vi "(Depricated) Poll Stepper Enable.vi"(8 "error in (no error)":errorcluster, 11 "cRIO-CO2 in":refnum<class "cRIO-CO2.lvclass">) -> (0 "error out":errorcluster, 3 "cRIO-CO2 out":refnum<class "cRIO-CO2.lvclass">)   [LabVIEW 2015]
uses:
  cRIO-CO2 Messages/Launch Stepper Msg/Launch Syringe Stepper Msg.lvclass
  cRIO-CO2.lvclass
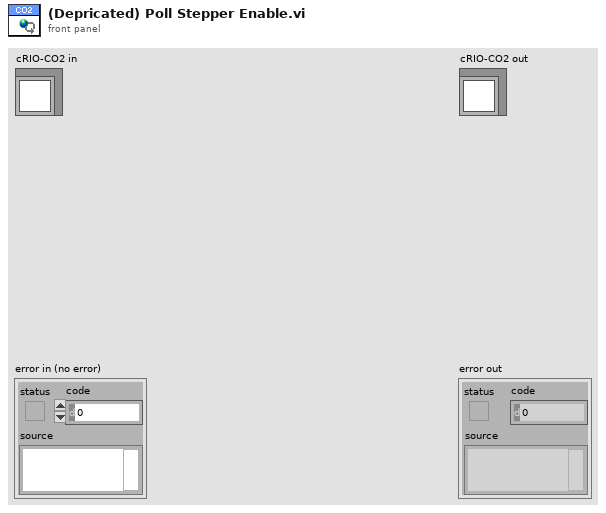
[diagram p1: front panel]
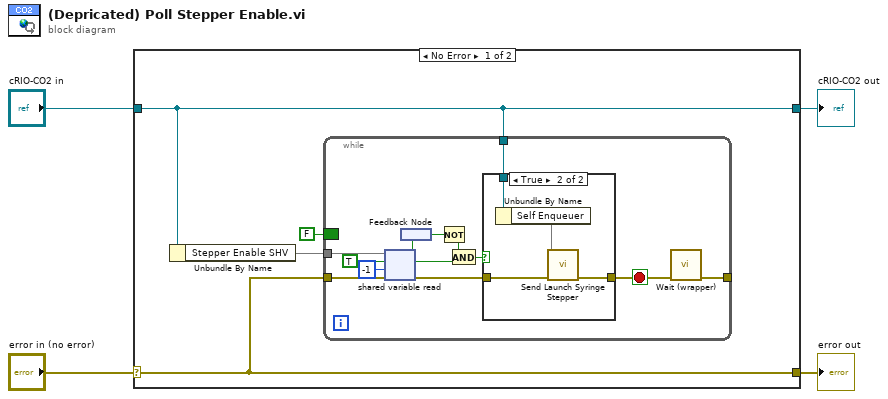
[diagram p0: block diagram]
diagram:
  n1 = case shown="No Error" "error in (no error)" {
    selector: "error in (no error)" -> [w7 w27]
    tunnel: [w7 w27] -> w3
    tunnel: [w6 w26] -> w1
    tunnel: "cRIO-CO2 in" -> [w6 w26]
    frame No Error {
      n2 = Unbundle By Name(w6) -> ("Stepper Enable SHV"=w8)
      n3 = while {
        tunnel: w8 -> [w18]
        tunnel: w7 -> [w17]
        border: FALSE -> [_]
        tunnel: w6 -> [w11]
        tunnel: [w9] -> _
        stop <- w10 stop-if-true
        n4 = shared-variable-read(w18, w17, TRUE, -1 ("timeout ms")) -> (w16:errorcluster, w15:bool)  [unwired: 3 out]
        n5 = feedback-in #1(w15) -> ()
        n6 = feedback #1() -> (w14:bool)
        n7 = Not(x=w14) -> (.not. x?=w13:bool)
        n8 = And(x=w13, y=w15) -> (x .and. y?=w12:bool)
        n9 = case shown="True" w12 {
          tunnel: w16 -> [w21 w25]
          tunnel: [w21 w22] -> w10
          tunnel: w11 -> [_ w24]
          frame False {
          }
          frame True {
            n10 = Unbundle By Name(w24) -> ("Self Enqueuer"=w23)
            n11 = call "Send Launch Syringe Stepper.vi"("error in (no error)"=w25, "Message Enqueuer"=w23) -> ("error out"=w22:errorcluster)  [unwired: 8 in, 1 out]
          }
        }
        n12 = call "Wait (wrapper).vi"("error in (no error)"=w10) -> ("error out"=w9:errorcluster)  [unwired: 10 in]
      }
    }
    frame Error {
    }
  }
  "error out" <- w3
  "cRIO-CO2 out" <- w1
